vi "load_class.vi"(8 "error in (no error)":errorcluster, 10 "class_path":path, 11 "class":refnum<class "v1.lvclass">) -> (0 "error out":errorcluster)   [LabVIEW 2015, in "lv-dialog.lvlib" / "v1.lvlib"]
uses:
  v1.lvlib
  v1.lvclass
  private/_controls/fg_command.ctl
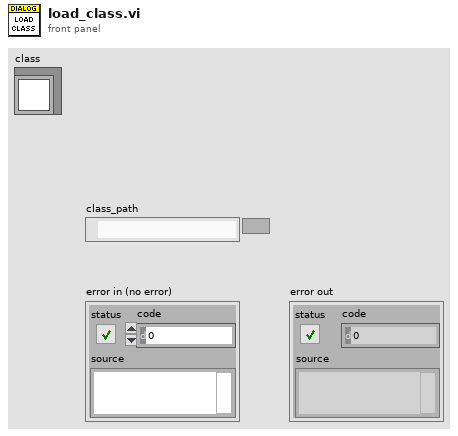
[diagram p1: front panel]
types:
  T1 = typedef "lv-dialog.lvlib/v1.lvlib/fg_command.ctl" = enum16{"null", "initialize", "read", "write", "shutdown"}
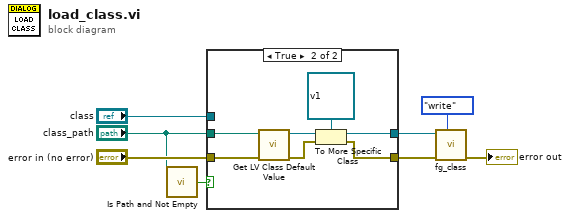
[diagram p0: block diagram]
diagram:
  n1 = call <vilib>:"Is Path and Not Empty.vi"("path"="class_path") -> ("Is Path and Not Empty?"=w3:bool)  [unwired: 4 in]
  n2 = case shown="True" w3 {
    tunnel: "error in (no error)" -> [w9 w17]
    tunnel: [w10 w13] -> w7
    tunnel: [w9 w12] -> w6
    tunnel: "class_path" -> [_ w11]
    tunnel: "class" -> [w10 _]
    frame False {
    }
    frame True {
      n3 = call <vilib>:"Get LV Class Default Value.vi"("error in (no error)"=w17, "class path"=w11) -> ("error out"=w15:errorcluster, "object"=w16:refnum<class>)  [unwired: 8 in]
      n4 = To More Specific Class(target class=refnum<class "v1.lvclass"> refnum ("lv-dialog.lvlib:v1.lvclass"), reference=w16, error in=w15) -> (specific class reference=w13:refnum<class "v1.lvclass">, error out=w12:errorcluster)
    }
  }
  n5 = call "fg_class.vi"("fg_command"=fg_command."write", "error in (no error)"=w6, "class in"=w7) -> ("error out"=→"error out":errorcluster)  [unwired: 7 in, 1 out]
